vi "file output directory.vi"(8 "error in":errorcluster) -> (0 "error out":errorcluster, 2 "exists":bool, 3 "data directory":path)   [LabVIEW 2017]
uses:
  <vilib>/Utility/sysdir.llb/System Directory Type.ctl
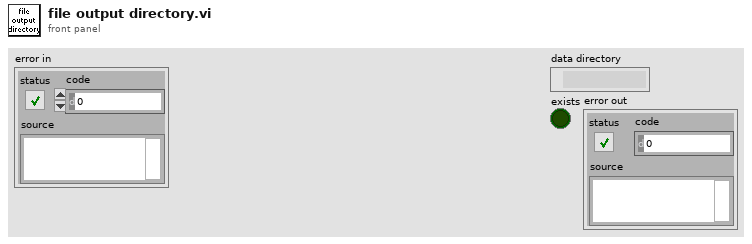
[diagram p1: front panel]
types:
  T1 = typedef "System Directory Type.ctl" = i32
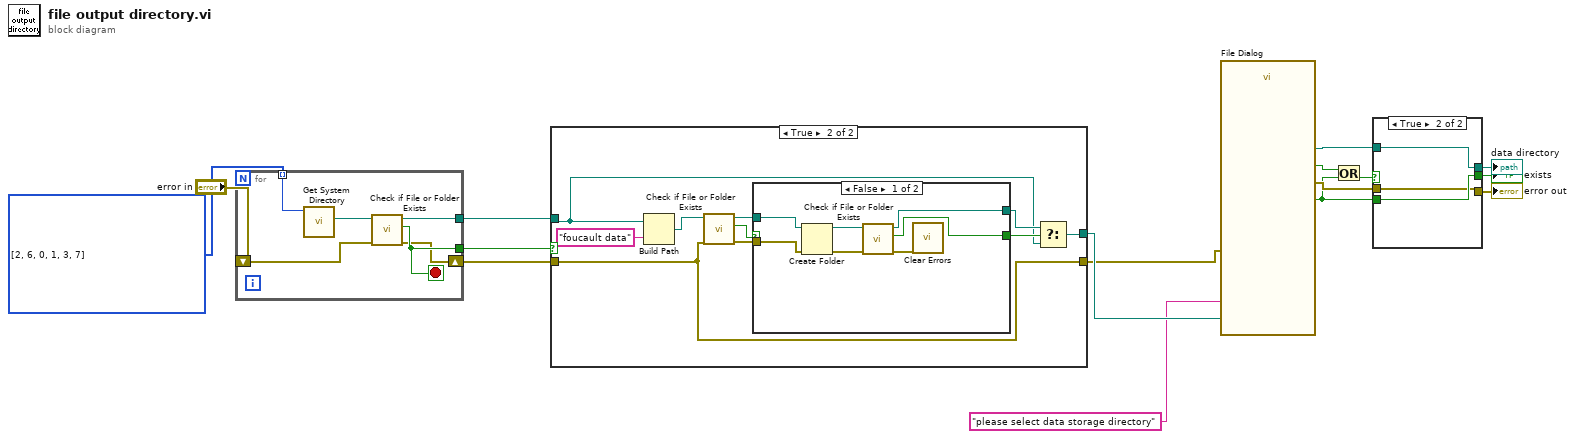
[diagram p0: block diagram]
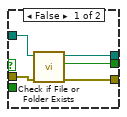
[diagram p2: hidden frame]
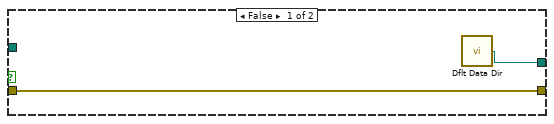
[diagram p3: hidden frame]
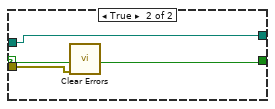
[diagram p4: hidden frame]
diagram:
  w16 = T1[] [2, 6, 0, 1, 3, 7] items=["User Home"=0, "User Desktop"=1, "User Documents"=2, "User Application Data"=3, "User Preferences"=4, "User Temporary"=5, "Public Documents"=6, "Public Application Data"=7, "Public Preferences"=8, "Public Cache"=13, "System Core Libraries"=9, "System Installed Libraries"=10, "Application Files"=11, "Boot Volume Root"=12] ("Array")
  n1 = for {
    tunnel: w16 -> [w21] mode=indexing
    tunnel: [w20] -> w15
    tunnel: [w19] -> w14
    shift-right: [w18] -> w13
    shift-left: "error in" -> [w17]
    stop <- w20 stop-if-true
    n2 = call <vilib>:"Get System Directory.vi"("system directory type"=w21) -> ("system directory"=w22:path)  [unwired: 10 in]
    n3 = call <vilib>:"Check if File or Folder Exists.vi"("error in (no error)"=w17, "path"=w22) -> ("error out"=w18:errorcluster, "file or folder exists?"=w20:bool, "dup path"=w19:path)  [unwired: 7 in]
  }
  n4 = case shown="True" w15 {
    tunnel: w14 -> [_ w27]
    tunnel: w13 -> [w23 w25]
    tunnel: [w24 w26] -> w11
    tunnel: [w23 w25] -> w9
    frame False {
      n5 = call <vilib>:"Dflt Data Dir.vi"() -> ("App:Default Data Directory"=w24:path)
    }
    frame True {
      n6 = Build Path(base path=w27, name or relative path="foucault data") -> (appended path=w33:path)
      n7 = call <vilib>:"Check if File or Folder Exists.vi"("error in (no error)"=w25, "path"=w33) -> ("error out"=w31:errorcluster, "file or folder exists?"=w30:bool, "dup path"=w32:path)  [unwired: 7 in]
      n8 = case shown="False" w30 {
        selector: w30 -> [_ w44]
        tunnel: w32 -> [w41 w43]
        tunnel: w31 -> [w40 w42]
        tunnel: [w36 w44] -> w29
        tunnel: [w35 w43] -> w28
        frame False {
          n9 = Create Folder(path (use dialog)=w41, error in=w40) -> (created path=w39:path, error out=w38:errorcluster)  [unwired: 1 in, 1 out]
          n10 = call <vilib>:"Check if File or Folder Exists.vi"("error in (no error)"=w38, "path"=w39) -> ("error out"=w37:errorcluster, "file or folder exists?"=w36:bool, "dup path"=w35:path)  [unwired: 7 in]
          n11 = call <vilib>:"Clear Errors.vi"("error in (no error)"=w37) -> ()  [unwired: 5 in, 2 out]
        }
        frame True {
          n12 = call <vilib>:"Clear Errors.vi"("error in (no error)"=w42) -> ()  [unwired: 5 in, 2 out]
        }
      }
      n13 = Select(t=w28, s=w29, f=w27) -> (s? t:f=w26:path)
    }
  }
  n14 = call "File Dialog"("start path"=w11, "prompt"="please select data storage directory", "error in"=w9) -> ("selected path"=w8:path, "exists"=w4:bool, "cancelled"=w5:bool, "error out"=w7:errorcluster)  [unwired: 9 in]
  n15 = Or(x=w5, y=w4) -> (x .or. y?=w6:bool)
  n16 = case shown="True" w6 {
    tunnel: w8 -> [w49 w51]
    tunnel: w7 -> [w48 w50]
    tunnel: [w47 w51] -> w3
    tunnel: [w46 w52] -> w2
    tunnel: [w45 w50] -> w1
    tunnel: w4 -> [_ w52]
    frame False {
      n17 = call <vilib>:"Check if File or Folder Exists.vi"("error in (no error)"=w48, "path"=w49) -> ("error out"=w45:errorcluster, "file or folder exists?"=w46:bool, "dup path"=w47:path)  [unwired: 7 in]
    }
    frame True {
    }
  }
  "data directory" <- w3
  "exists" <- w2
  "error out" <- w1
